vi "Log API.vi"(7 "priority (normal)":T1, 8 "error in (no error)":T2, 10 "data":string, 11 "message":string(combo)) -> (0 "error out":T2)   [LabVIEW 2019, in "Log.lvlib"]
uses:
  Log.lvlib
  <vilib>/event_ctls.llb/usereventprio.ctl
  log module message.ctl
  Log GV.vi
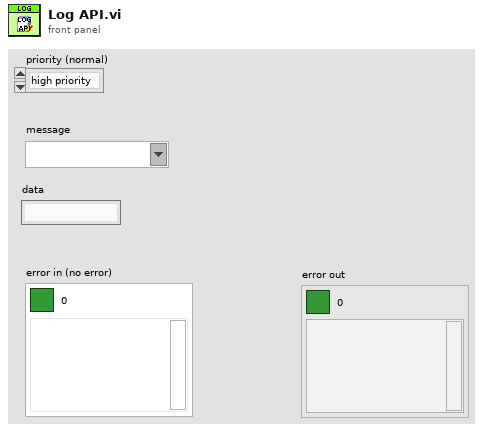
[diagram p1: front panel]
types:
  T1 = typedef "usereventprio.ctl" = enum32{"high priority", "normal priority"}
  T2 = cluster{"Boolean Round":bool, "code":i32, "source":string}
  T3 = typedef "Log.lvlib/log module message.ctl" = cluster{"msg":string, "data":string}
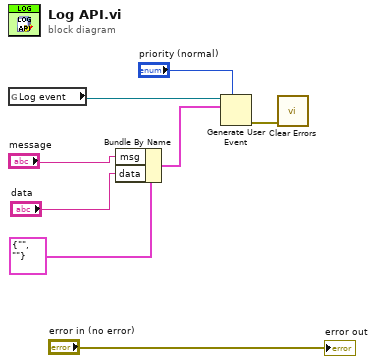
[diagram p0: block diagram]
diagram:
  n1 = global read "Log GV.vi" "Log event"() -> (w8:refnum<user-event>)
  n2 = Bundle By Name(cluster=T3 {"msg"="", "data"=""} ("Log message"), "msg"="message", "data"="data") -> (w5:T3)
  n3 = Generate User Event(priority (normal)="priority (normal)", user event=w8, event data cluster=w5) -> (error out=w4:errorcluster)  [unwired: 1 in, 1 out]
  n4 = call <vilib>:"Clear Errors.vi"("error in (no error)"=w4) -> ()  [unwired: 5 in, 2 out]
  "error out" <- "error in (no error)"
